vi "Critical Data Variable.vi"() -> ()   [LabVIEW 2010]
panel:
  in  "Critical Data":dbl[](array[numeric])
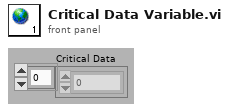
[diagram p1: front panel]
diagram:
